vi "DriveSetRobotStartingOrientationDeg.vi"(11 "GyroIntDirection":dbl) -> ()   [LabVIEW 2023]
doc: "set GyroIntDir\n\nIn;uts\n-- GyroIntdir -- Double -- This is the direction the robot is facing when the match starts. It is relative to the \n DRIVER (degrees)"
uses:
  DriveGlobal.vi
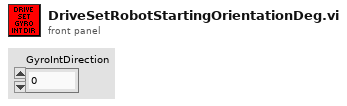
[diagram p1: front panel]
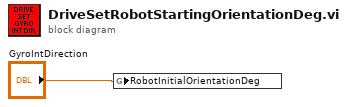
[diagram p0: block diagram]
diagram:
  n1 = global write "DriveGlobal.vi" "RobotInitialOrientationDeg"("GyroIntDirection") -> ()
